vi "BehaviorID.vi"() -> ()   [LabVIEW 2011]
panel:
  in  "Behavior":dbl
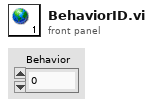
[diagram p1: front panel]
diagram:
